vi "formulaNode陣列測試.vi"() -> ()   [LabVIEW 2015]
panel:
  out "Line Data":cluster{"X":sgl, "Y":sgl, "T":sgl}
  out "cluster":cluster{"X":i32, "Y":i32}
  out "ClustArray":cluster{"X":i32, "Y":i32}[](array[cluster])
  out "2D ClustArray":i32[][](array[numeric])
  out "1D ClustArray":i32[](array[numeric])=[1, 2, 3, 4, 5, 0, 0, 0, 0, 0, 0, 0, 0, 0, 0, 0, 0, 0, 0, 0]
  out "2D Array":i32[][](array[numeric])
  out "1D Array":i32[](array[numeric])=[1, 2, 3, 4, 5, 0, 0, 0, 0, 0, 0, 0, 0, 0, 0, 0, 0, 0, 0, 0]
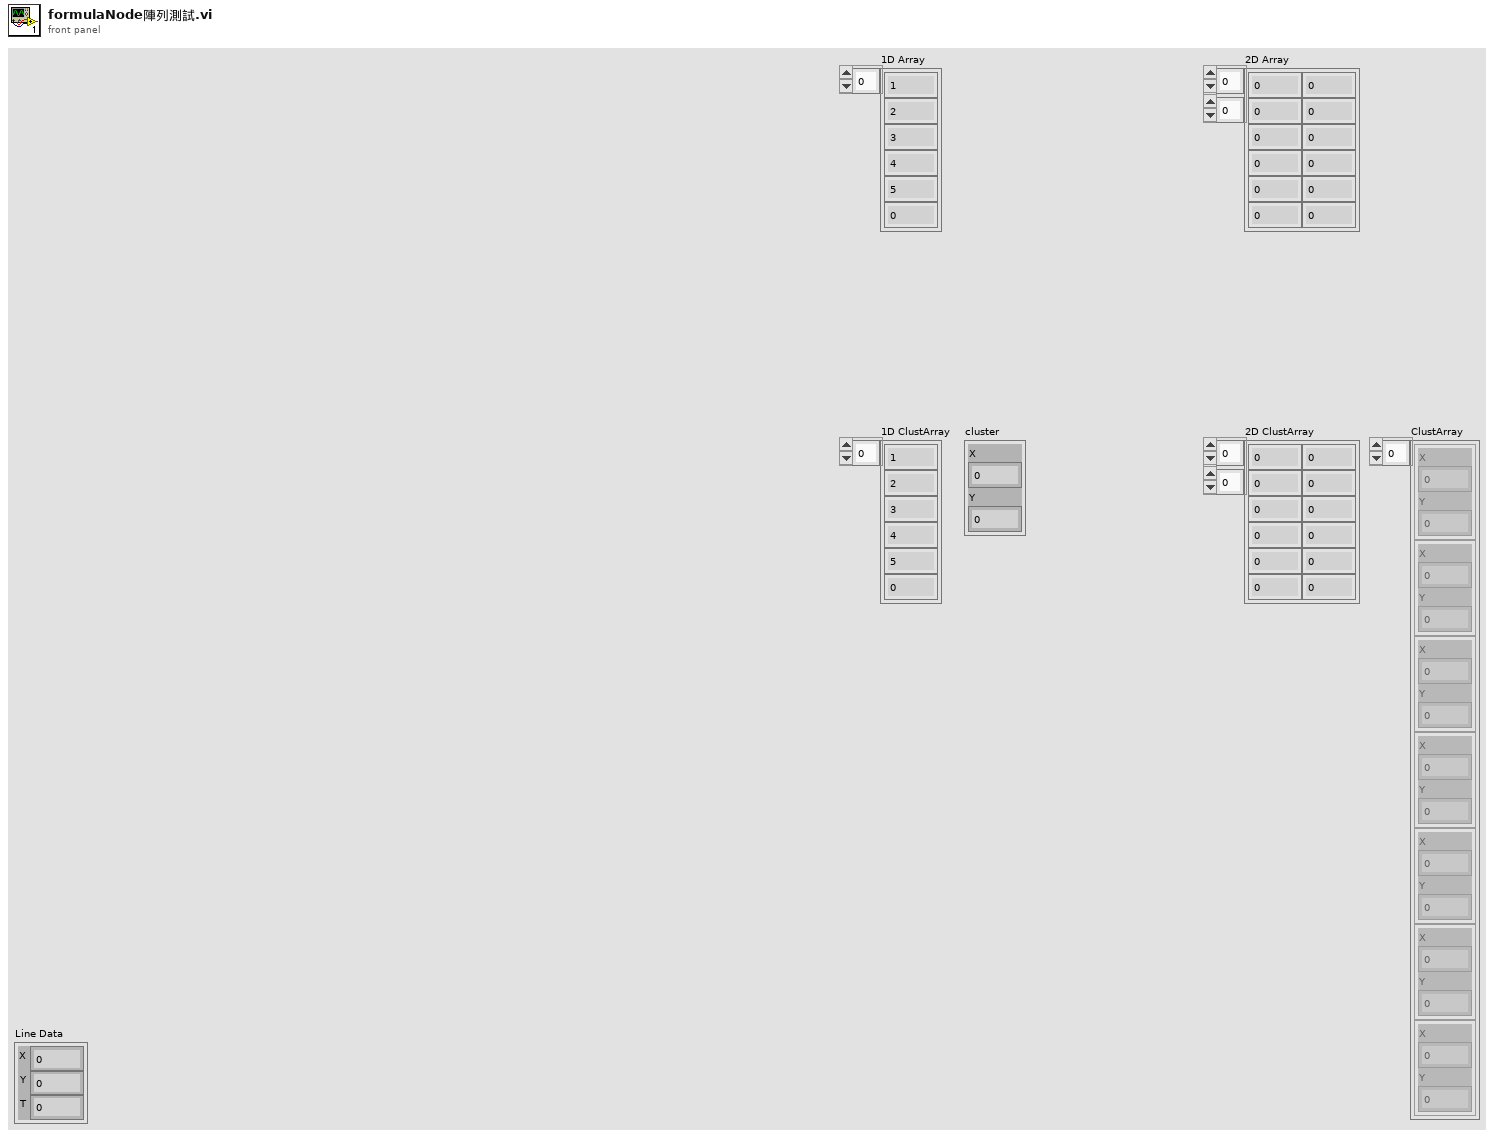
[diagram p1: front panel]
types:
  T1 = cluster{"Point 1":cluster{"X":sgl, "Y":sgl}, "Point 2":cluster{"X":sgl, "Y":sgl}}
  T2 = cluster{"center_X":dbl, "center_Y":dbl, "rotate":dbl}
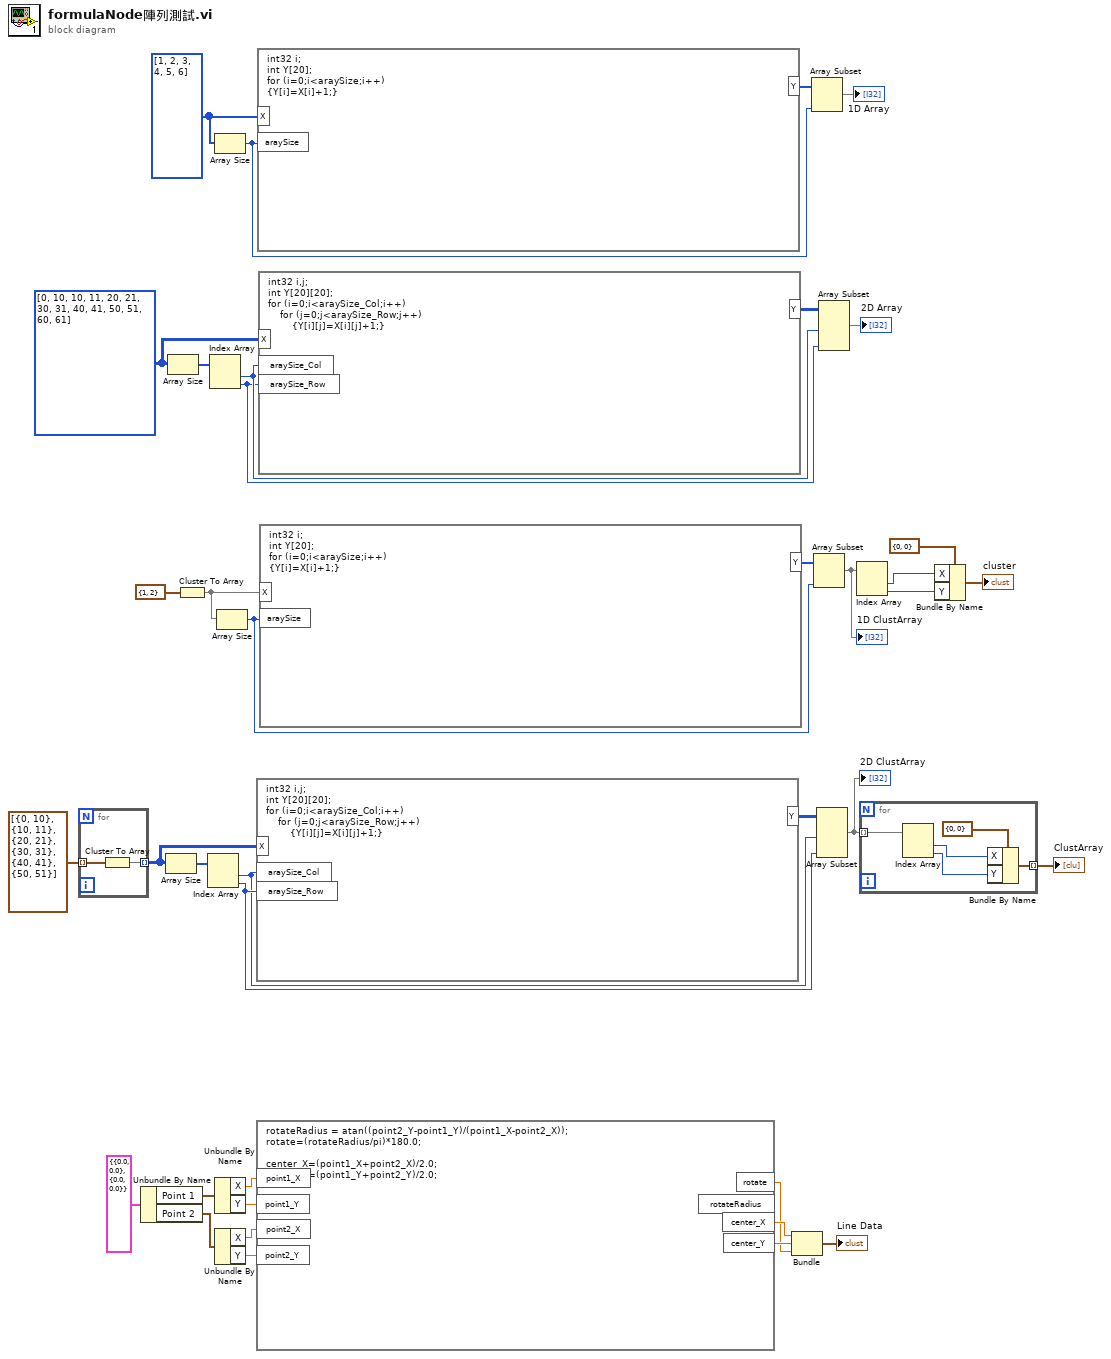
[diagram p0: block diagram]
diagram:
  w34 = i32[][] [[0, 10], [10, 11], [20, 21], [30, 31], [40, 41], [50, 51], [60, 61]]
  w38 = i32[] [1, 2, 3, 4, 5, 6]
  n1 = for {
    tunnel: cluster{i32, i32}[] [{0, 10}, {10, 11}, {20, 21}, {30, 31}, {40, 41}, {50, 51}] -> [w40] mode=indexing
    tunnel: [w39] -> w22 mode=indexing
    n2 = Cluster To Array(cluster=w40) -> (array=w39:i32[])
  }
  n3 = Unbundle By Name(T1 {"Point 1"={"X"=0.0, "Y"=0.0}, "Point 2"={"X"=0.0, "Y"=0.0}} ("input cluster")) -> ("Point 1"=w10:cluster{"X":sgl, "Y":sgl}, "Point 2"=w11:cluster{"X":sgl, "Y":sgl})
  n4 = Array Size(array=w22) -> (size(s)=w23:i32[])
  n5 = Array Size(array=w34) -> (size(s)=w33:i32[])
  n6 = Cluster To Array(cluster=cluster{"X":i32, "Y":i32} {"X"=1, "Y"=2}) -> (array=w26:i32[])
  n7 = Index Array(array=w23) -> (element #1=w19:i32, element #2=w20:i32)  [unwired: 2 in]
  n8 = Index Array(array=w33) -> (element #1=w30:i32, element #2=w29:i32)  [unwired: 2 in]
  n9 = Array Size(array=w38) -> (size(s)=w36:i32)
  n10 = Unbundle By Name(w10) -> ("X"=w8:sgl, "Y"=w7:sgl)
  n11 = Unbundle By Name(w11) -> ("X"=w6:sgl, "Y"=w5:sgl)
  n12 = Array Size(array=w26) -> (size(s)=w27:i32)
  n13 = formula code="int32 i,j;\nint Y[20][20];\nfor (i=0;i<araySize_Col;i++)\n    for (j=0;j<araySize_Row;j++)\n        {Y[i][j]=X[i][j]+1;}"("X"=w22, "araySize_Col"=w19, "araySize_Row"=w20) -> ("Y"=w24:i32[][])
  n14 = formula code="rotateRadius = atan((point2_Y-point1_Y)/(point1_X-point2_X));\nrotate=(rotateRadius/pi)*180.0;\n\ncenter_X=(point1_X+point2_X)/2.0;\ncenter_Y=(point1_Y+point2_Y)/2.0;"("point1_X"=w8, "point1_Y"=w7, "point2_X"=w6, "point2_Y"=w5) -> ("rotate"=w2:dbl, "center_X"=w4:dbl, "center_Y"=w3:dbl)  [unwired: 1 out]
  n15 = formula code="int32 i;\nint Y[20];\nfor (i=0;i<araySize;i++)\n{Y[i]=X[i]+1;}"("X"=w38, "araySize"=w36) -> ("Y"=w37:i32[])
  n16 = formula code="int32 i,j;\nint Y[20][20];\nfor (i=0;i<araySize_Col;i++)\n    for (j=0;j<araySize_Row;j++)\n        {Y[i][j]=X[i][j]+1;}"("X"=w34, "araySize_Col"=w30, "araySize_Row"=w29) -> ("Y"=w32:i32[][])
  n17 = formula code="int32 i;\nint Y[20];\nfor (i=0;i<araySize;i++)\n{Y[i]=X[i]+1;}"("X"=w26, "araySize"=w27) -> ("Y"=w28:i32[])
  n18 = Bundle("center_X"=w4, "center_Y"=w3, "rotate"=w2) -> (→"Line Data":T2)  [unwired: 1 in]
  n19 = Array Subset(array=w37, length=w36) -> (→"1D Array":i32[])  [unwired: 1 in]
  n20 = Array Subset(array=w28, length=w27) -> (w17:i32[])  [unwired: 1 in]
  "1D ClustArray" <- w17
  n21 = Array Subset(array=w24, length (row)=w19, length (col)=w20) -> (w21:i32[][])  [unwired: 2 in]
  "2D ClustArray" <- w21
  n22 = Array Subset(array=w32, length (row)=w30, length (col)=w29) -> (→"2D Array":i32[][])  [unwired: 2 in]
  n23 = Index Array(array=w17) -> (element #1=w15:i32, element #2=w14:i32)  [unwired: 2 in]
  n24 = for {
    tunnel: w21 -> [w45] mode=indexing
    tunnel: [w44] -> w18 mode=indexing
    n25 = Index Array(array=w45) -> (element #1=w42:i32, element #2=w41:i32)  [unwired: 2 in]
    n26 = Bundle By Name(cluster=cluster{"X":i32, "Y":i32} {"X"=0, "Y"=0}, "X"=w42, "Y"=w41) -> (w44:cluster{"X":i32, "Y":i32})
  }
  "ClustArray" <- w18
  n27 = Bundle By Name(cluster=cluster{"X":i32, "Y":i32} {"X"=0, "Y"=0}, "X"=w15, "Y"=w14) -> (→"cluster":cluster{"X":i32, "Y":i32})
